vi "TestComSpeed.vi"(8 "error in (no error)":errorcluster, 10 "Channel":i32, 11 "ID In":i32) -> (0 "error out":errorcluster, 1 "spd_rcvt":i32, 2 "code":i32, 3 "ID Out":i32, 4 "spd_kernel":i32)   [LabVIEW 2022 SP3, in "EClib functions.lvlib"]
uses:
  EClib functions.lvlib
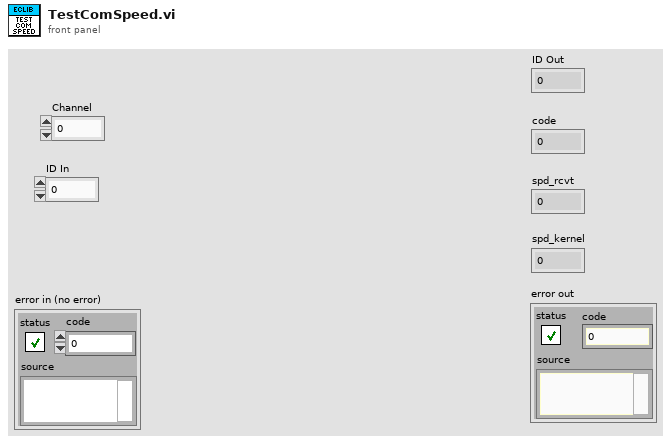
[diagram p1: front panel]
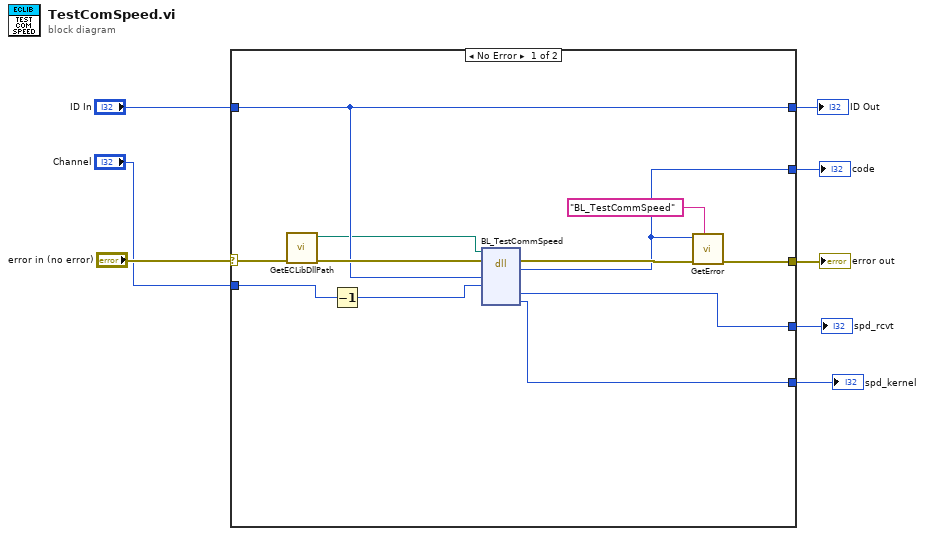
[diagram p0: block diagram]
diagram:
  n1 = case shown="No Error" "error in (no error)" {
    selector: "error in (no error)" -> [w20 w21]
    tunnel: [w13 w21] -> w5
    tunnel: "ID In" -> [w18 w22]
    tunnel: [w18 w22] -> w8
    tunnel: [w12 _] -> w4
    tunnel: [w16 _] -> w3
    tunnel: [w15 _] -> w2
    tunnel: "Channel" -> [w10 _]
    frame No Error {
      n2 = call "GetECLibDllPath.vi"("error in (no error)"=w20) -> ("error out"=w19:errorcluster, "ECLibDLLPath"=w17:path)  [unwired: 9 in]
      n3 = Decrement(x=w10) -> (x-1=w9:i32)
      n4 = dll-call lib="C:/EC-Lab Development Package/EC-Lab Development Package/EClib.dll" fn="BL_TestCommSpeed"(path in=w17, error in=w19, "ID"=w18, "channel"=w9) -> (error out=w14:errorcluster, "return type"=w12:i32, "spd_rcvt"=w16:i32, "spd_kernel"=w15:i32)  [unwired: 5 in, 1 out]
      n5 = call "GetError.vi"("DLLFunction"="BL_TestCommSpeed", "error in"=w14, "code"=w12) -> ("error out"=w13:errorcluster)  [unwired: 8 in]
    }
    frame Error {
    }
  }
  "error out" <- w5
  "ID Out" <- w8
  "code" <- w4
  "spd_rcvt" <- w3
  "spd_kernel" <- w2
